vi "Gen_TrajLib_Doc_Macros.vi"() -> ()   [LabVIEW 2019]
doc: "Generates and HTML file with the Description of every class, library, ctl, and vi in every open project. Creates separate documents for each library and virtual folder , and links to the top level document. In addition, for every VI shows connector pane. Saves the HTML file in folder <project folder>\\<project name> Documentation\\Documentation.html. erases previous content if any. \nDoes not create documentation for Documentation folder in project if exists. Does not create documentation for packed libraries in the project."
uses:
  Doc_Builder_SubVI/FileAndPath.ctl
  <vilib>/Utility/NIReport.llb/NI_report.lvclass
panel:
  out "Full Library Path":path
  out "Current Section":string
  out "File Index":i32
  out "File Count":i32
  in  "stop":bool
  out "Full Input File Name":path
  in  "GO":bool
  in  "Documentation Path":path=path "../HTML_Build_Work/Temp"
  in  "Library Path":path=path "../../FRC_LV_Trajectory_Library/Macros"
  out "Full Doc Path":path
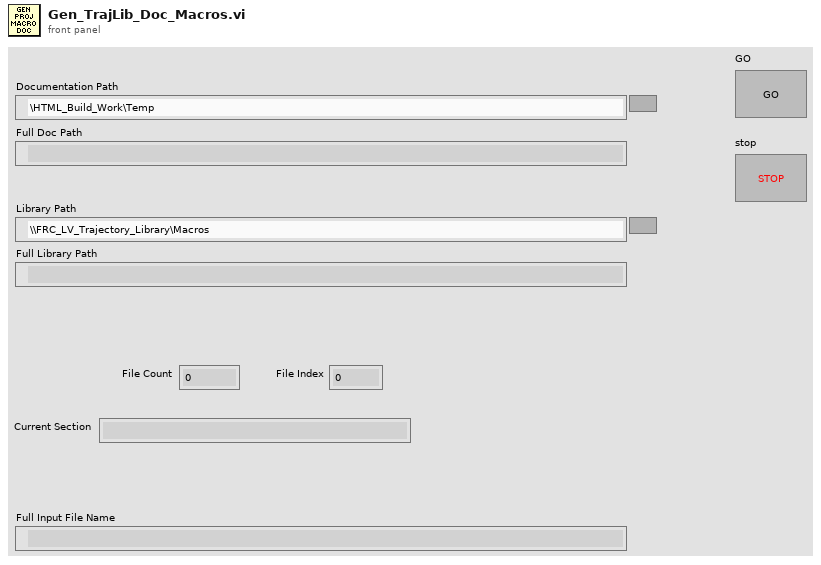
[diagram p1: front panel]
types:
  T1 = typedef "FileAndPath.ctl" = cluster{"FileName":string, "Library Path":path}
  T2 = enum16{"Standard Report", "HTML", "Word", "Excel"}
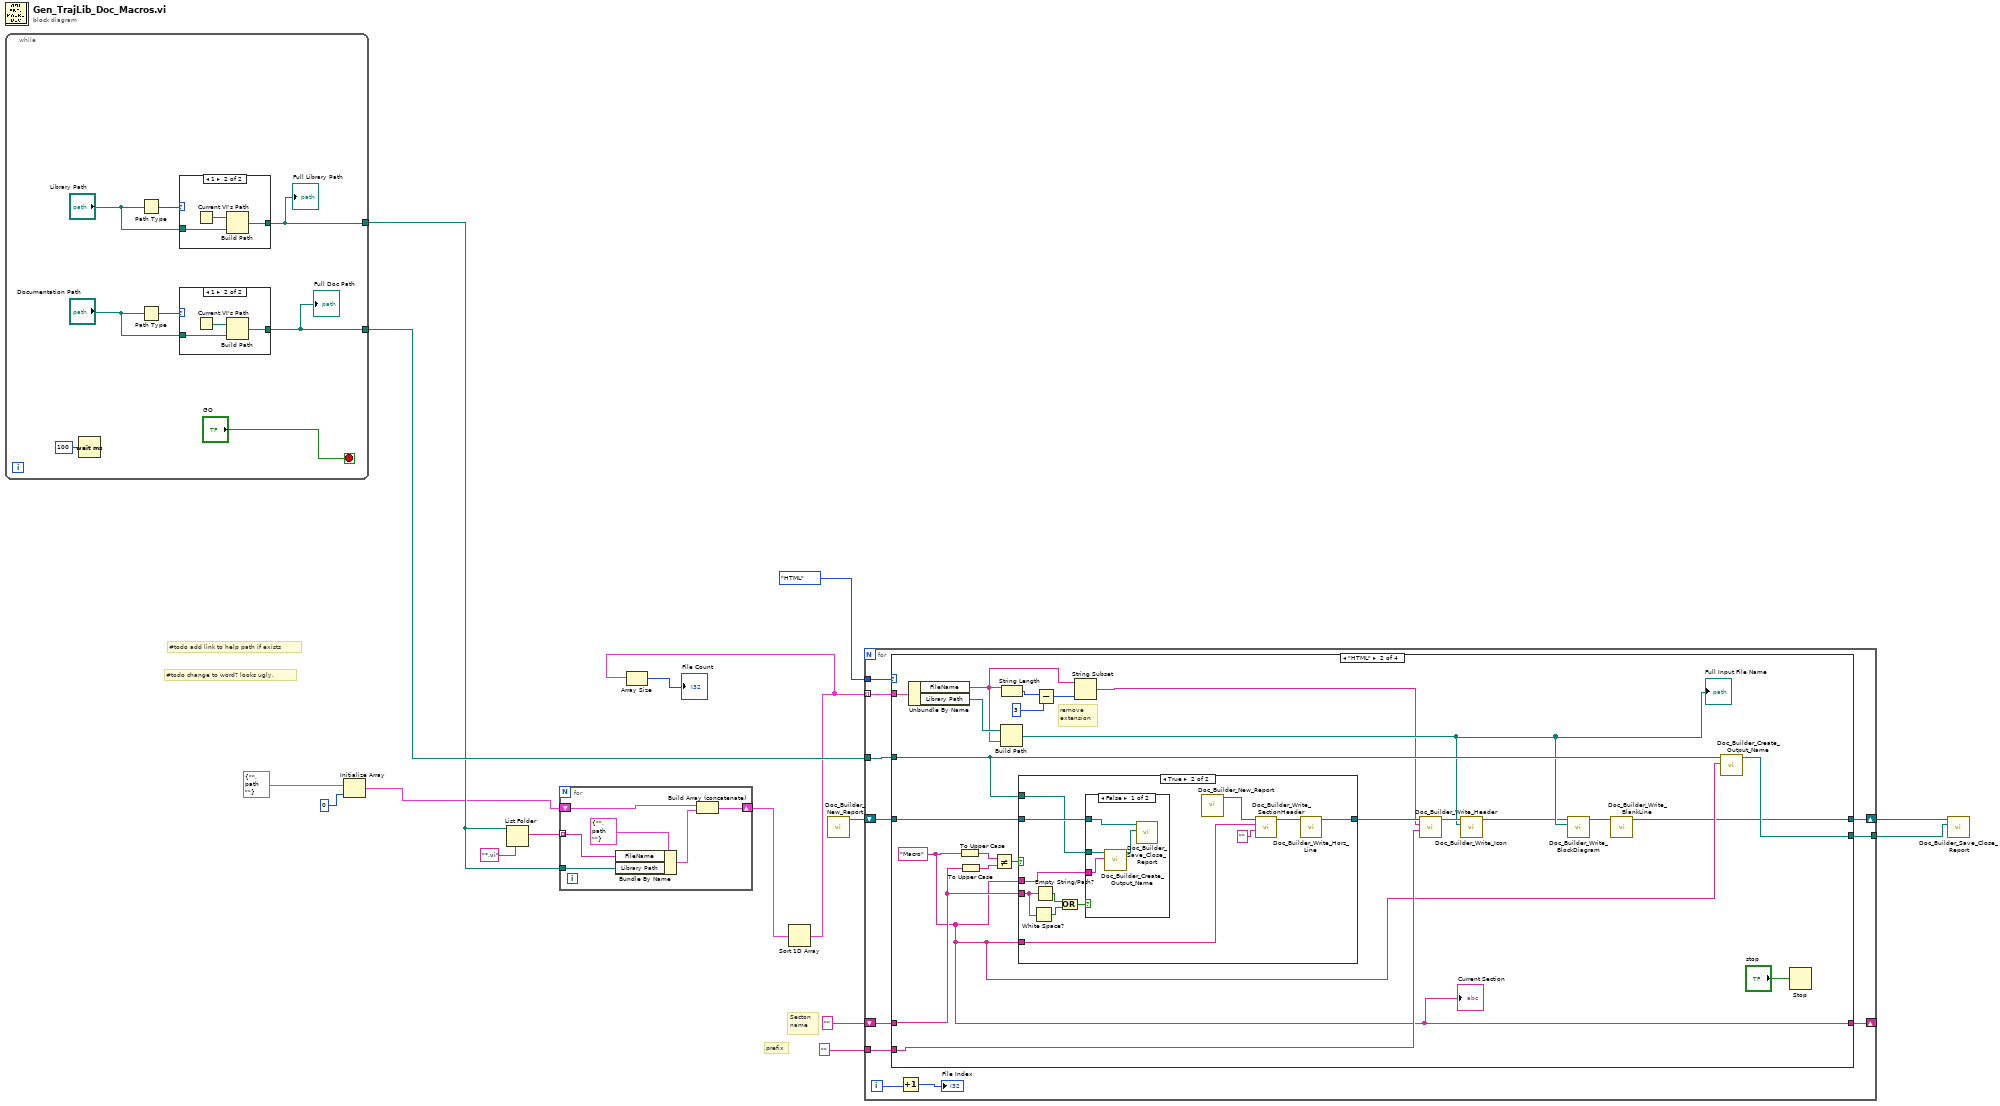
[diagram p0: block diagram]
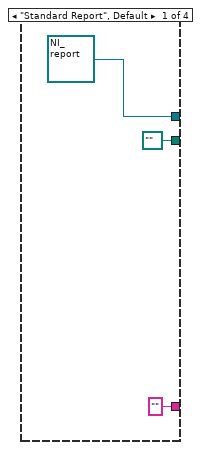
[diagram p4: hidden frame]
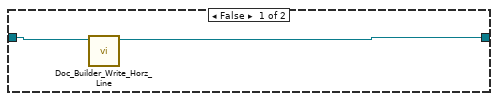
[diagram p5: hidden frame]
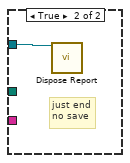
[diagram p6: hidden frame]
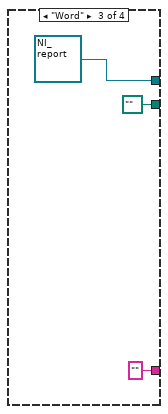
[diagram p7: hidden frame]
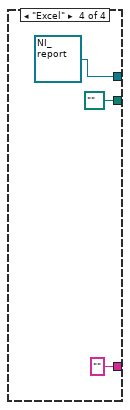
[diagram p8: hidden frame]
diagram:
  # "Secton \nname"
  # "prefix"
  # "#todo change to word? looks ugly."
  # "#todo add link to help path if exists"
  n1 = while {
    tunnel: [w18] -> w14
    tunnel: [w17] -> w10
    stop <- "GO" stop-if-true
    n2 = Wait (ms)(milliseconds to wait=u32 100) -> ()  [unwired: 1 out]
    n3 = Path Type(1:"Library Path") -> (0:w21:i16)
    n4 = Path Type(1:"Documentation Path") -> (0:w22:i16)
    n5 = case shown="1" w21 {
      tunnel: [w25 w27] -> w17
      tunnel: "Library Path" -> [w25 w26]
      frame 0, Default {
      }
      frame 1 {
        n6 = Current VI's Path() -> (path=w28:path)
        n7 = Build Path(base path=w28, name or relative path=w26) -> (appended path=w27:path)
      }
    }
    "Full Library Path" <- w17
    n8 = case shown="1" w22 {
      tunnel: [w29 w31] -> w18
      tunnel: "Documentation Path" -> [w29 w30]
      frame 0, Default {
      }
      frame 1 {
        n9 = Current VI's Path() -> (path=w32:path)
        n10 = Build Path(base path=w32, name or relative path=w30) -> (appended path=w31:path)
      }
    }
    "Full Doc Path" <- w18
  }
  n11 = Initialize Array(T1 {"FileName"="", "Library Path"=path ""} ("FileAndPath"), 0 ("dimension size")) -> (w8:T1[])
  n12 = List Folder(path=w10, pattern="*.vi") -> (filenames=w11:string[])  [unwired: 2 in, 3 out]
  n13 = for {
    tunnel: w11 -> [w38] mode=indexing
    tunnel: w10 -> [w37]
    shift-right: [w36] -> w1
    shift-left: w8 -> [w35]
    n14 = Bundle By Name(cluster=T1 {"FileName"="", "Library Path"=path ""} ("FileAndPath"), "FileName"=w38, "Library Path"=w37) -> (w33:T1)
    n15 = Build Array (concatenate)(w35, w33) -> (w36:T1[])
  }
  n16 = Sort 1D Array(array=w1) -> (sorted array=w6:T1[])
  n17 = Array Size(array=w6) -> (size(s)=→"File Count":i32)
  n18 = call "Doc_Builder_New_Report.vi"() -> ("NI_report out"=w5:refnum<class "NI_report.lvclass">)  [unwired: 11 in]
  n19 = for {
    tunnel: w6 -> [w48] mode=indexing
    tunnel: T2."HTML" ("report type") -> [w49]
    tunnel: w14 -> [w47]
    tunnel: "" ("string") -> [w44]
    shift-right: [w40] -> w3
    shift-left: w5 -> [w43]
    shift-right: [w39] -> _
    shift-left: "" ("string") -> [w42]
    tunnel: [w41] -> w2
    i -> [w46]
    n20 = case shown="\"HTML\"" w49 {
      tunnel: w48 -> [_ w70 _ _]
      tunnel: w47 -> [_ w61 _ _]
      tunnel: w44 -> [_ w59 _ _]
      tunnel: w43 -> [_ w65 _ _]
      tunnel: w42 -> [_ w62 _ _]
      tunnel: [path "" ("Full Report Name") w63 path "" ("Full Report Name") path "" ("Full Report Name")] -> w41
      tunnel: [refnum<class "NI_report.lvclass"> refnum ("report out") w55 refnum<class "NI_report.lvclass"> refnum ("report out") refnum<class "NI_report.lvclass"> refnum ("report out")] -> w40
      tunnel: ["" ("FileName") w57 "" ("FileName") "" ("FileName")] -> w39
      frame "Standard Report", Default {
      }
      frame "HTML" {
        w57 = "Macro" ("string")
        # "remove\nextension"
        n21 = Unbundle By Name(w70) -> ("FileName"=w68:string, "Library Path"=w69:path)
        n22 = To Upper Case(1:w57) -> (0:w67:string)
        n23 = To Upper Case(1:w62) -> (0:w66:string)
        n24 = Not Equal?(x=w67, y=w66) -> (x != y?=w58:bool)
        n25 = Build Path(base path=w69, name or relative path=w68) -> (appended path=w60:path)
        "Full Input File Name" <- w60
        n26 = String Length(string=w68) -> (length=w74:i32)
        n27 = case shown="True" w58 {
          tunnel: w65 -> [w77 w86]
          tunnel: [w76 w83] -> w64
          tunnel: w62 -> [_ w84]
          tunnel: w61 -> [_ w85]
          tunnel: w57 -> [_ w80]
          tunnel: w57 -> [_ w79]
          frame False {
            n28 = call "Doc_Builder_Write_Horz_Line.vi"("NI_report in"=w77) -> ("NI_report out"=w76:refnum<class "NI_report.lvclass">)  [unwired: 10 in]
          }
          frame True {
            n29 = White Space?(1:w84) -> (0:w88:bool)
            n30 = Empty String/Path?(string/path=w84) -> (empty?=w87:bool)
            n31 = Or(x=w87, y=w88) -> (x .or. y?=w89:bool)
            n32 = case shown="False" w89 {
              tunnel: w86 -> [w93 w94]
              tunnel: w85 -> [w92 _]
              tunnel: w79 -> [w91 _]
              frame False {
                n33 = call "Doc_Builder_Create_Output_Name.vi"("Section Name"=w91, "Path"=w92) -> ("Full Report Name"=w90:path)  [unwired: 9 in]
                n34 = call "Doc_Builder_Save_Close_Report.vi"("appended path"=w90, "NI_report in"=w93) -> ()  [unwired: 9 in, 1 out]
              }
              frame True {
                # "just end\nno save"
                n35 = call-dynamic "Dispose Report.vi"("report in"=w94) -> ()  [unwired: 14 in, 1 out]
              }
            }
            n36 = call "Doc_Builder_New_Report.vi"() -> ("NI_report out"=w82:refnum<class "NI_report.lvclass">)  [unwired: 11 in]
            n37 = call "Doc_Builder_Write_SectionHeader.vi"("Prefix String"="", "Section Name"=w80, "NI_report in"=w82) -> ("NI_report out"=w81:refnum<class "NI_report.lvclass">)  [unwired: 8 in]
            n38 = call "Doc_Builder_Write_Horz_Line.vi"("NI_report in"=w81) -> ("NI_report out"=w83:refnum<class "NI_report.lvclass">)  [unwired: 10 in]
          }
        }
        n39 = Subtract(x=w74, y=3) -> (x-y=w72:i32)
        n40 = String Subset(string=w68, length (rest)=w72) -> (substring=w53:string)  [unwired: 1 in]
        n41 = call "Doc_Builder_Write_Header.vi"("Prefix String"=w59, "Item Name"=w53, "NI_report in"=w64) -> ("NI_report out"=w71:refnum<class "NI_report.lvclass">)  [unwired: 8 in]
        n42 = call "Doc_Builder_Write_Icon.vi"("Input Item file path"=w60, "NI_report in"=w71) -> ("NI_report out"=w54:refnum<class "NI_report.lvclass">)  [unwired: 9 in]
        n43 = call "Doc_Builder_Write_BlockDiagram.vi"("input item file path"=w60, "NI_report in"=w54) -> ("NI_report out"=w56:refnum<class "NI_report.lvclass">)  [unwired: 9 in]
        n44 = call "Doc_Builder_Write_BlankLine.vi"("NI_report in"=w56) -> ("NI_report out"=w55:refnum<class "NI_report.lvclass">)  [unwired: 10 in]
        n45 = call "Doc_Builder_Create_Output_Name.vi"("Section Name"=w57, "Path"=w61) -> ("Full Report Name"=w63:path)  [unwired: 9 in]
        n46 = Stop(stop? (T)="stop") -> ()
        "Current Section" <- w57
      }
      frame "Word" {
      }
      frame "Excel" {
      }
    }
    n47 = Increment(x=w46) -> (x+1=→"File Index":i32)
  }
  n48 = call "Doc_Builder_Save_Close_Report.vi"("appended path"=w2, "NI_report in"=w3) -> ()  [unwired: 9 in, 1 out]
